vi "RT Driver VI.vi"(7 "Operation":T1, 11 "Device Reference in":T2 format="%.0x") -> (0 "Error Code":i32)   [LabVIEW 2020, in "Communication Bus Template Engine.lvlib"]
uses:
  Communication Bus Template Engine.lvlib
  <vilib>/NI/NIVS Inline Async API/_VS Inline Async API/VS Inline Async API/VS Inline Async API.lvclass
  <vilib>/NI VeriStand/Custom Device API/Custom Device API.lvlib
  <vilib>/NI VeriStand/Custom Device API/Get Item Property (Variant).vi
  Shared/Compiled.Settings.ctl
  Shared/Communication Bus Template Shared.lvlib
  Shared/Constants.vi
  <vilib>/NI VeriStand/Custom Device Tools/Custom Device Utility Library/Custom Device Utility Library.lvlib
  <vilib>/NI VeriStand/Custom Device API/Data Reference.ctl
  <vilib>/NI VeriStand/Custom Device API/Block Data Reference.ctl
  Shared/Execution Unit Compiled Information.ctl
  Includes/Communication Bus Interfaces.lvlibp/Execution Unit/Execution Unit/Execution Unit.lvclass
  Execution Unit Runtime Information.ctl
  RTStateVariables.ctl
  <vilib>/NI VeriStand/Custom Device API/Custom Device Item Ref.ctl
  <vilib>/NI VeriStand/Custom Device API/Hardware Interface Driver VI Operation.ctl
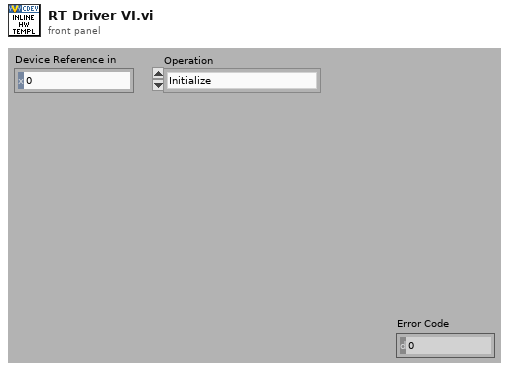
[diagram p1: front panel]
types:
  T1 = typedef "Custom Device API.lvlib/Hardware Interface Driver VI Operation.ctl" = enum16{"Initialize", "Start", "Read Data from HW", "Write Data to HW", "Close"}
  T2 = typedef "Custom Device API.lvlib/Custom Device Item Ref.ctl" = u64
  T3 = typedef "Communication Bus Template Engine.lvlib/RTStateVariables.ctl" = cluster{"Async":refnum<class "VS Inline Async API.lvclass">, "Execution Unit Runtime Information":T4}
  T4 = typedef "Communication Bus Template Engine.lvlib/Execution Unit Runtime Information.ctl" = cluster{"Execution Unit":refnum<class "Execution Unit.lvclass">, "Incoming Buffer":dbl[], "Outgoing Buffer":dbl[], "Incoming Data References":T5[], "Outgoing Data References":T6[]}
  T5 = typedef "Custom Device API.lvlib/Data Reference.ctl" = i32
  T6 = typedef "Custom Device API.lvlib/Block Data Reference.ctl" = cluster{"Data Reference":T5, "Offset":u64, "Length":u64}
  T7 = typedef "Communication Bus Template Shared.lvlib/Compiled.Settings.ctl" = cluster{"Name":string, "Execution Unit Compiled Information":T8}
  T8 = typedef "Communication Bus Template Shared.lvlib/Execution Unit Compiled Information.ctl" = cluster{"Flattened Execution Unit":string, "Incoming Buffer":dbl[], "Outgoing Buffer":dbl[], "Incoming Data References":T5[], "Outgoing Data References":T6[]}
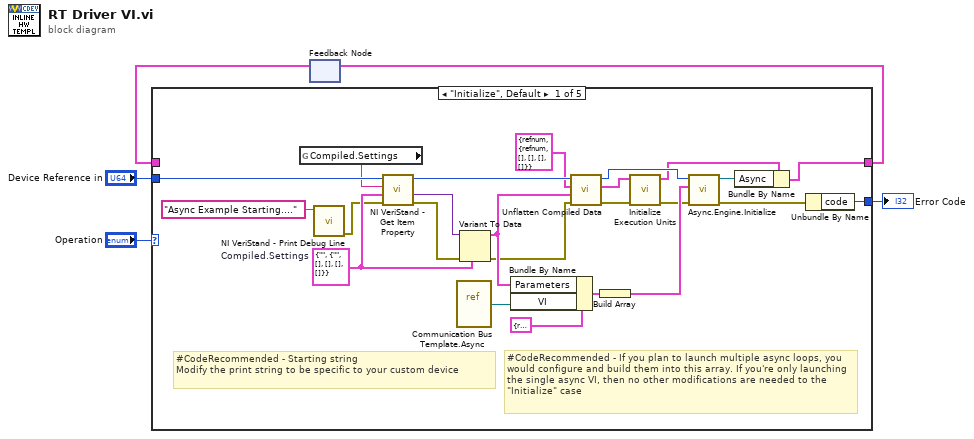
[diagram p0: block diagram]
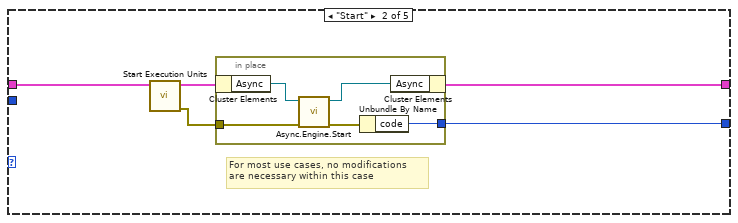
[diagram p2: hidden frame]
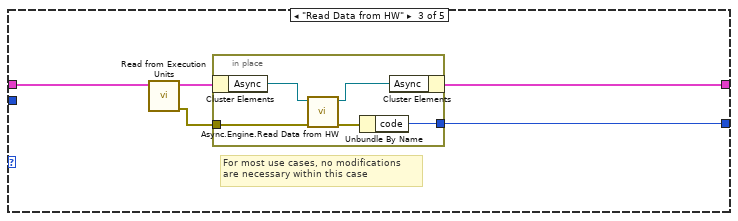
[diagram p3: hidden frame]
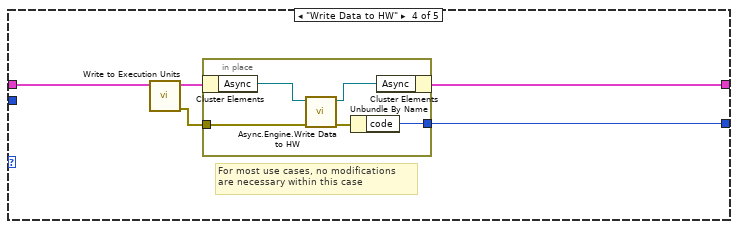
[diagram p4: hidden frame]
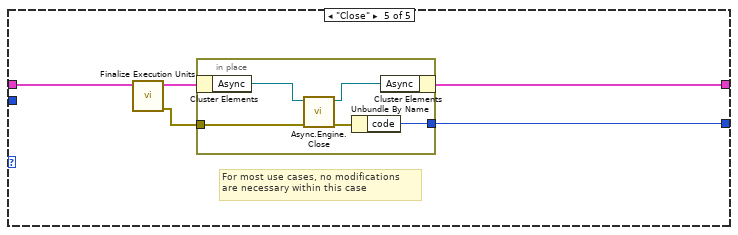
[diagram p5: hidden frame]
diagram:
  n1 = feedback #1() -> (w3:T3)  [unwired: 1 out]
  n2 = case shown="\"Initialize\", Default" "Operation" {
    tunnel: [w15 w33 w43 w53 w63] -> w4
    tunnel: w3 -> [_ w34 w42 w52 w64]
    tunnel: "Device Reference in" -> [w25 _ _ _ _]
    tunnel: [w29 w32 w44 w54 w62] -> w1
    frame "Initialize", Default {
      w21 = T7 {"Name"="", "Execution Unit Compiled Information"={"Flattened Execution Unit"="", "Incoming Buffer"=[], "Outgoing Buffer"=[], "Incoming Data References"=[], "Outgoing Data References"=[]}}  # Compiled.Settings
      # "#CodeRecommended - Starting string\nModify the print string to be specific to your custom device"
      # "#CodeRecommended - If you plan to launch multiple async loops, you would configure and build them into this array. If you're only launching the single async VI, then no other modifications are needed to the \"Initialize\" case"
      n3 = global read "Constants.vi" "Compiled.Settings"() -> (w22:string)
      n4 = call <vilib>:"NI VeriStand - Print Debug Line.vi"("Message"="Async Example Starting....") -> ("error out"=w19:errorcluster)  [unwired: 10 in]
      n5 = call-poly <vilib>:"NI VeriStand - Get Item Property.vi"("error in (no error)"=w19, "Default Value"=w21, "Property Name"=w22, "Item Ref in"=w25) -> ("error out"=w24:errorcluster, "Value"=w23:variant, "Item Ref out"=w10:T2)  [unwired: 4 in, 1 out]
      n6 = vi-ref "Communication Bus Template.Async.vi"() -> (w17:refnum<vi>)
      n7 = Variant To Data(error in=w24, type=w21, Variant=w23) -> (data=w14:T7, error out=w13:errorcluster)
      n8 = Bundle By Name(cluster=cluster{"VI":refnum<vi>, "Parameters":variant} {"VI"=refnum, "Parameters"=variant} ("Process"), "Parameters"=w14, "VI"=w17) -> (w26:cluster{"VI":refnum<vi>, "Parameters":variant})
      n9 = call "Unflatten Compiled Data.vi"("error in (no error)"=w13, "Compiled.Settings"=w14, "RT State Variables in"=T3 {"Async"=refnum, "Execution Unit Runtime Information"={"Execution Unit"=refnum, "Incoming Buffer"=[], "Outgoing Buffer"=[], "Incoming Data References"=[], "Outgoing Data References"=[]}}, "Item Ref in"=w10) -> ("error out"=w12:errorcluster, "RT State Variables out"=w7:T3, "Item Ref out"=w11:T2)  [unwired: 5 in]
      n10 = Build Array(w26) -> (w20:cluster{"VI":refnum<vi>, "Parameters":variant}[])
      n11 = call "Initialize Execution Units.vi"("error in (no error)"=w12, "RT State Variables in"=w7) -> ("error out"=w8:errorcluster, "RT State Variables out"=w6:T3)  [unwired: 8 in]
      n12 = call <vilib>:"Async.Engine.Initialize.vi"("error in (no error)"=w8, "Processes"=w20, "Custom Device Ref"=w11) -> ("error out"=w16:errorcluster, "Async"=w28:refnum<class "VS Inline Async API.lvclass">)  [unwired: 7 in]
      n13 = Bundle By Name(cluster=w6, "Async"=w28) -> (w15:T3)
      n14 = Unbundle By Name(w16) -> ("code"=w29:i32)
    }
    frame "Start" {
      # "For most use cases, no modifications \nare necessary within this case"
      n15 = call "Start Execution Units.vi"("RT State Variables in"=w34) -> ("error out"=w30:errorcluster, "RT State Variables out"=w31:T3)  [unwired: 9 in]
      n16 = in-place {
        in-place-border: [w36] -> w32
        in-place-border: w30 -> [w35]
        n17 = in-place-cluster #2(w31) -> ("Async"=w39:refnum<class "VS Inline Async API.lvclass">)
        n18 = call <vilib>:"Async.Engine.Start.vi"("error in (no error)"=w35, "VS Inline Async API in"=w39) -> ("error out"=w37:errorcluster, "VS Inline Async API out"=w38:refnum<class "VS Inline Async API.lvclass">)  [unwired: 8 in]
        n19 = Unbundle By Name(w37) -> ("code"=w36:i32)
        n20 = in-place-cluster #2("Async"=w38) -> (w33:T3)
      }
    }
    frame "Read Data from HW" {
      # "For most use cases, no modifications \nare necessary within this case"
      n21 = call "Read from Execution Units.vi"("RT State Variables in"=w42) -> ("error out"=w40:errorcluster, "RT State Variables out"=w41:T3)  [unwired: 9 in]
      n22 = in-place {
        in-place-border: [w47] -> w44
        in-place-border: w40 -> [w45]
        n23 = in-place-cluster #3(w41) -> ("Async"=w49:refnum<class "VS Inline Async API.lvclass">)
        n24 = call <vilib>:"Async.Engine.Read Data from HW.vi"("error in"=w45, "Async in"=w49) -> ("error out"=w46:errorcluster, "Async out"=w48:refnum<class "VS Inline Async API.lvclass">)  [unwired: 8 in]
        n25 = Unbundle By Name(w46) -> ("code"=w47:i32)
        n26 = in-place-cluster #3("Async"=w48) -> (w43:T3)
      }
    }
    frame "Write Data to HW" {
      # "For most use cases, no modifications \nare necessary within this case"
      n27 = call "Write to Execution Units.vi"("RT State Variables in"=w52) -> ("error out"=w50:errorcluster, "RT State Variables out"=w51:T3)  [unwired: 9 in]
      n28 = in-place {
        in-place-border: [w59] -> w54
        in-place-border: w50 -> [w55]
        n29 = in-place-cluster #4(w51) -> ("Async"=w57:refnum<class "VS Inline Async API.lvclass">)
        n30 = call <vilib>:"Async.Engine.Write Data to HW.vi"("error in (no error)"=w55, "VS Inline Async API in"=w57) -> ("error out"=w58:errorcluster, "VS Inline Async API out"=w56:refnum<class "VS Inline Async API.lvclass">)  [unwired: 8 in]
        n31 = Unbundle By Name(w58) -> ("code"=w59:i32)
        n32 = in-place-cluster #4("Async"=w56) -> (w53:T3)
      }
    }
    frame "Close" {
      # "For most use cases, no modifications \nare necessary within this case"
      n33 = call "Finalize Execution Units.vi"("RT State Variables in"=w64) -> ("error out"=w60:errorcluster, "RT State Variables out"=w61:T3)  [unwired: 9 in]
      n34 = in-place {
        in-place-border: [w67] -> w62
        in-place-border: w60 -> [w65]
        n35 = in-place-cluster #5(w61) -> ("Async"=w69:refnum<class "VS Inline Async API.lvclass">)
        n36 = call <vilib>:"Async.Engine.Close.vi"("error in (no error)"=w65, "Async in"=w69) -> ("error out"=w66:errorcluster, "Async out"=w68:refnum<class "VS Inline Async API.lvclass">)  [unwired: 8 in]
        n37 = Unbundle By Name(w66) -> ("code"=w67:i32)
        n38 = in-place-cluster #5("Async"=w68) -> (w63:T3)
      }
    }
  }
  "Error Code" <- w1
  n39 = feedback-in #1(w4) -> ()
